vi "heinzingerControlGlobals.vi"() -> ()   [LabVIEW 2014]
uses:
  Controls/heinzingerSelect.ctl
panel:
  in  "postAccOffsetVoltState":T1
  in  "postAccOffsetVoltControl":T1
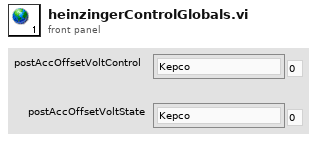
[diagram p1: front panel]
types:
  T1 = typedef "heinzingerSelect.ctl" = enum8{"Kepco", "Heinzinger0", "Heinzinger1", "Heinzinger2", "loading"}
diagram:
